vi "CTest.vi"() -> ()   [LabVIEW 2012]
uses:
  <vilib>/eio/EIONode/EIONode.xnode
  <vilib>/rvi/eio/common/nirviEmuTemplateMethod_errors.vi
panel:
  in  "stop":bool
  in  "Boolean 2":bool
  in  "Boolean":bool
  in  "Wait Time":i16
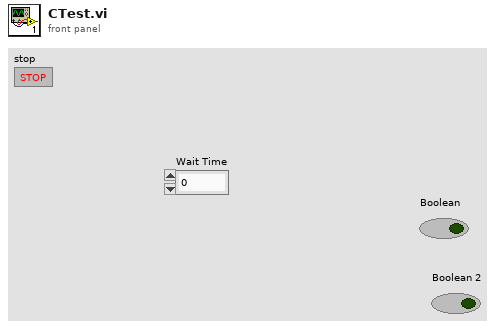
[diagram p1: front panel]
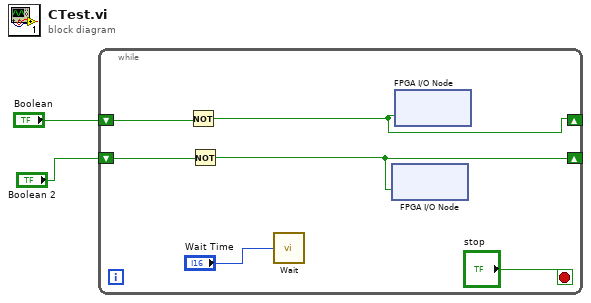
[diagram p0: block diagram]
diagram:
  n1 = while {
    shift-right: [w6] -> _
    shift-left: "Boolean 2" -> [w7]
    shift-right: [w4] -> _
    shift-left: "Boolean" -> [w5]
    stop <- "stop" stop-if-true
    n2 = Not(x=w5) -> (.not. x?=w4:bool)
    n3 = Not(x=w7) -> (.not. x?=w6:bool)
    n4 = call "Wait"("Count(uSec)"="Wait Time") -> ()  [unwired: 1 out]
    n5 = xnode "FPGA I/O Node"("DIO1"=w6) -> ()  [unwired: 1 in, 1 out]
    n6 = xnode "FPGA I/O Node"("DIO0"=w4) -> ()  [unwired: 1 in, 1 out]
  }
